vi "TIO Stream Write.vi"(7 "error in (no error)":errorcluster, 8 "Type":T1(ring)=enum."RPC Request", 9 "Payload":string, 10 "TC Connection":T2={"Type"=enum."Serial", "URL"="serial:///dev/cu.usbserial-00000", "TO"=500, "Addr"=0, "Port"=0, "TCP"=refnum, "UDP"=refnum, "Route"=""}) -> (0 "error out":errorcluster, 3 "TC Connection":T2={"Type"=enum."Serial", "URL"="serial:///dev/cu.usbserial-00000", "TO"=500, "Addr"=0, "Port"=0, "TCP"=refnum, "UDP"=refnum, "Route"=""})   [LabVIEW 2017]
uses:
  <instrlib>/tio-labview/TIO Library/TIO SLIP Encode.vi
  <instrlib>/tio-labview/TIO Library/TIO Serial Checksum CRC32.vi
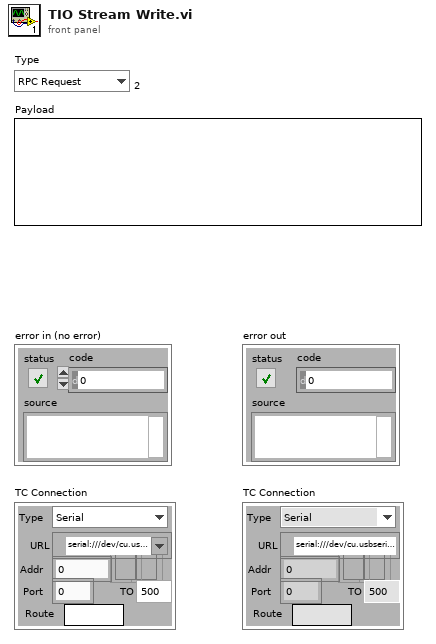
[diagram p1: front panel]
types:
  T1 = enum8{"Invalid", "Log", "RPC Request", "RPC Reply", "RPC Error", "Stream Description", "User"}
  T2 = cluster{"Type":enum16{"Serial", "TCP", "UDP", "mUDP"}, "URL":refnum<visa-resource-name>, "TO":u32, "Addr":u32, "Port":i32, "TCP":refnum<k5>, "UDP":refnum<k16>, "Route":string}
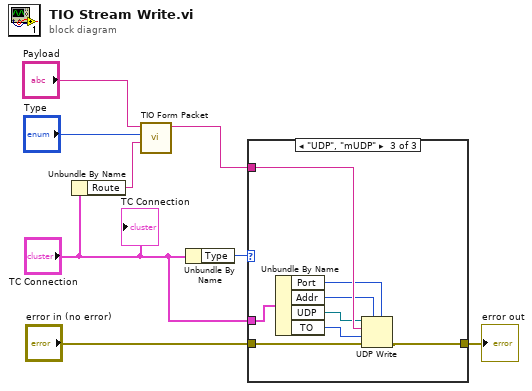
[diagram p0: block diagram]
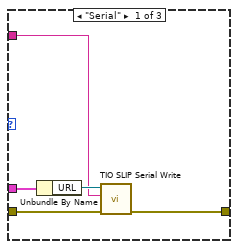
[diagram p2: hidden frame]
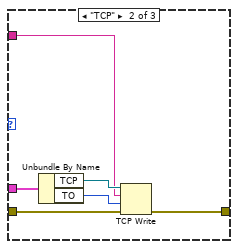
[diagram p3: hidden frame]
diagram:
  n1 = Unbundle By Name("TC Connection") -> ("Route"=w1:string)
  n2 = call <instrlib>:"TIO Form Packet.vi"("Routing"=w1, "Type"="Type", "Payload"="Payload") -> ("String out"=w4:string)  [unwired: 8 in]
  n3 = Unbundle By Name("TC Connection") -> ("Type"=w8:enum16{"Serial", "TCP", "UDP", "mUDP"})
  n4 = case shown="\"UDP\", \"mUDP\"" w8 {
    tunnel: w4 -> [w9 w14 w24]
    tunnel: "TC Connection" -> [w13 w19 w27]
    tunnel: "error in (no error)" -> [w11 w17 w26]
    tunnel: [w10 w15 w25] -> w6
    frame "Serial" {
      n5 = Unbundle By Name(w13) -> ("URL"=w12:refnum<visa-resource-name>)
      n6 = call <instrlib>:"TIO SLIP Serial Write.vi"("error in (no error)"=w11, "Data"=w9, "VISA Refnum in"=w12) -> ("error out"=w10:errorcluster)  [unwired: 8 in]
    }
    frame "TCP" {
      n7 = Unbundle By Name(w19) -> ("TCP"=w18:refnum<k5>, "TO"=w16:u32)
      n8 = TCP Write(connection ID=w18, data in=w14, error in (no error)=w17, 9:w16) -> (error out=w15:errorcluster)  [unwired: 2 out]
    }
    frame "UDP", "mUDP" {
      n9 = Unbundle By Name(w27) -> ("Port"=w20:i32, "Addr"=w21:u32, "UDP"=w23:refnum<k16>, "TO"=w22:u32)
      n10 = UDP Write(address=w21, port or service name=w20, connection ID=w23, data in=w24, 8:w26, 9:w22) -> (error out=w25:errorcluster)  [unwired: 1 out]
    }
  }
  "error out" <- w6
  "TC Connection" <- "TC Connection"
